vi "Write Address.vi"(8 "error in":errorcluster, 10 "Address":string, 11 "Alicat in":refnum<class "Alicat.lvclass">) -> (0 "error out":errorcluster, 3 "Alicat out":refnum<class "Alicat.lvclass">)   [LabVIEW 2014, in "Alicat.lvlib" / "Alicat.lvclass"]
uses:
  Alicat.lvclass
  Alicat.lvclass/Alicat.ctl
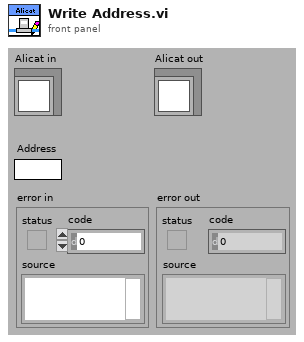
[diagram p1: front panel]
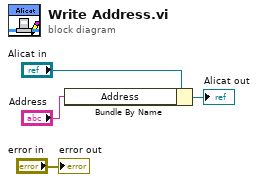
[diagram p0: block diagram]
diagram:
  n1 = Bundle By Name(cluster="Alicat in", "Address"="Address") -> (→"Alicat out":refnum<class "Alicat.lvclass">)
  "error out" <- "error in"
